vi "OscilloscopeDual.vi"() -> ()   [LabVIEW 2021]
uses:
  <userlib>/SciSDK/SciSDK_Labview.lvlib
panel:
  out "Digital CH3.3":i32[](graph)
  out "Digital CH3.2":i32[](graph)
  out "Digital CH3.1":i32[](graph)
  out "Digital CH3.0":i32[](graph)
  out "Digital CH2.3":i32[](graph)
  out "Digital CH2.2":i32[](graph)
  out "Digital CH2.1":i32[](graph)
  out "Digital CH2.0":i32[](graph)
  out "Digital CH1.3":i32[](graph)
  out "Digital CH1.2":i32[](graph)
  out "Digital CH1.1":i32[](graph)
  out "Digital CH1.0":i32[](graph)
  out "Digital CH0.3":i32[](graph)
  out "Digital CH0.2":i32[](graph)
  out "Digital CH0.1":i32[](graph)
  out "Analog CH1":dbl[](graph)
  out "Analog CH2":dbl[](graph)
  out "Analog CH3":dbl[](graph)
  out "Analog CH0":dbl[](graph)
  out "Digital CH0.0":i32[](graph)
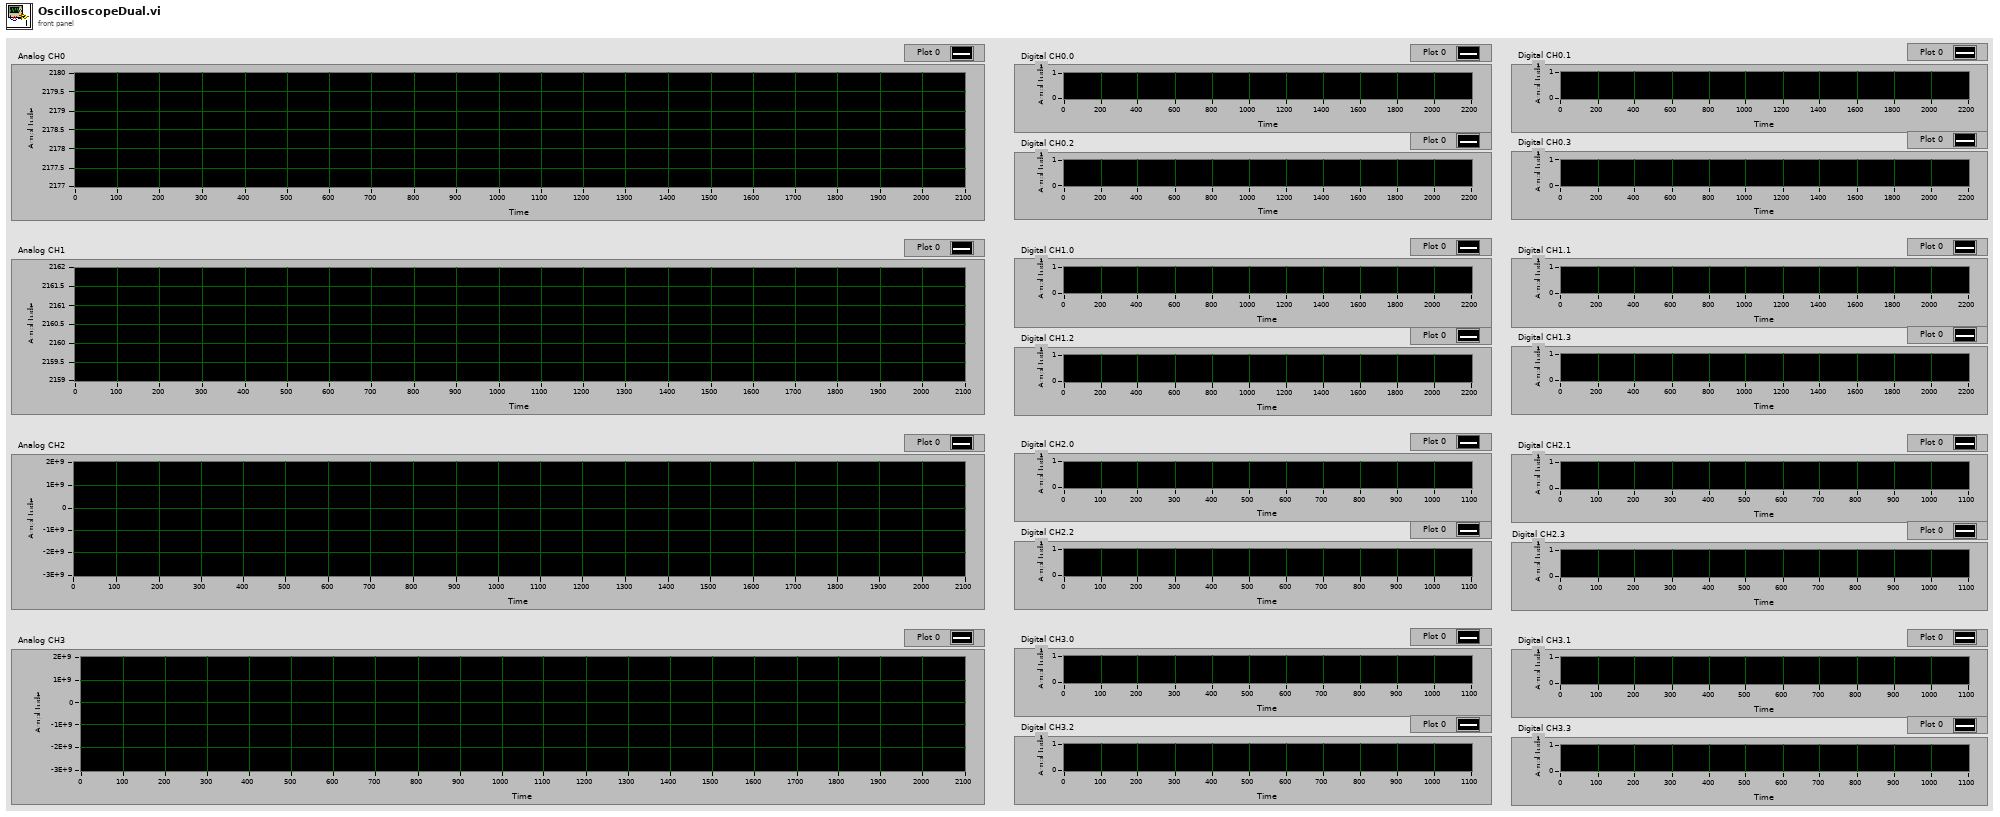
[diagram p1: front panel]
types:
  T1 = cluster{"Name":string, "Board Model":string, "Handle":u64}
  T2 = cluster{"Oscilloscope Dual Path":string, "Oscilloscope Dual Name":string}
  T3 = cluster{"Board Name":string, "Board Model":string, "Handle":u64}
  T4 = cluster{"magic":u32, "trigger_position":u32, "timecode":u32, "samples_analog":u32, "samples_digital":u32, "tracks_analog_per_channel":u32, "tracks_digital_per_channel":u32, "channels":u32, "analog":dbl[][], "digital_data":i32[][]}
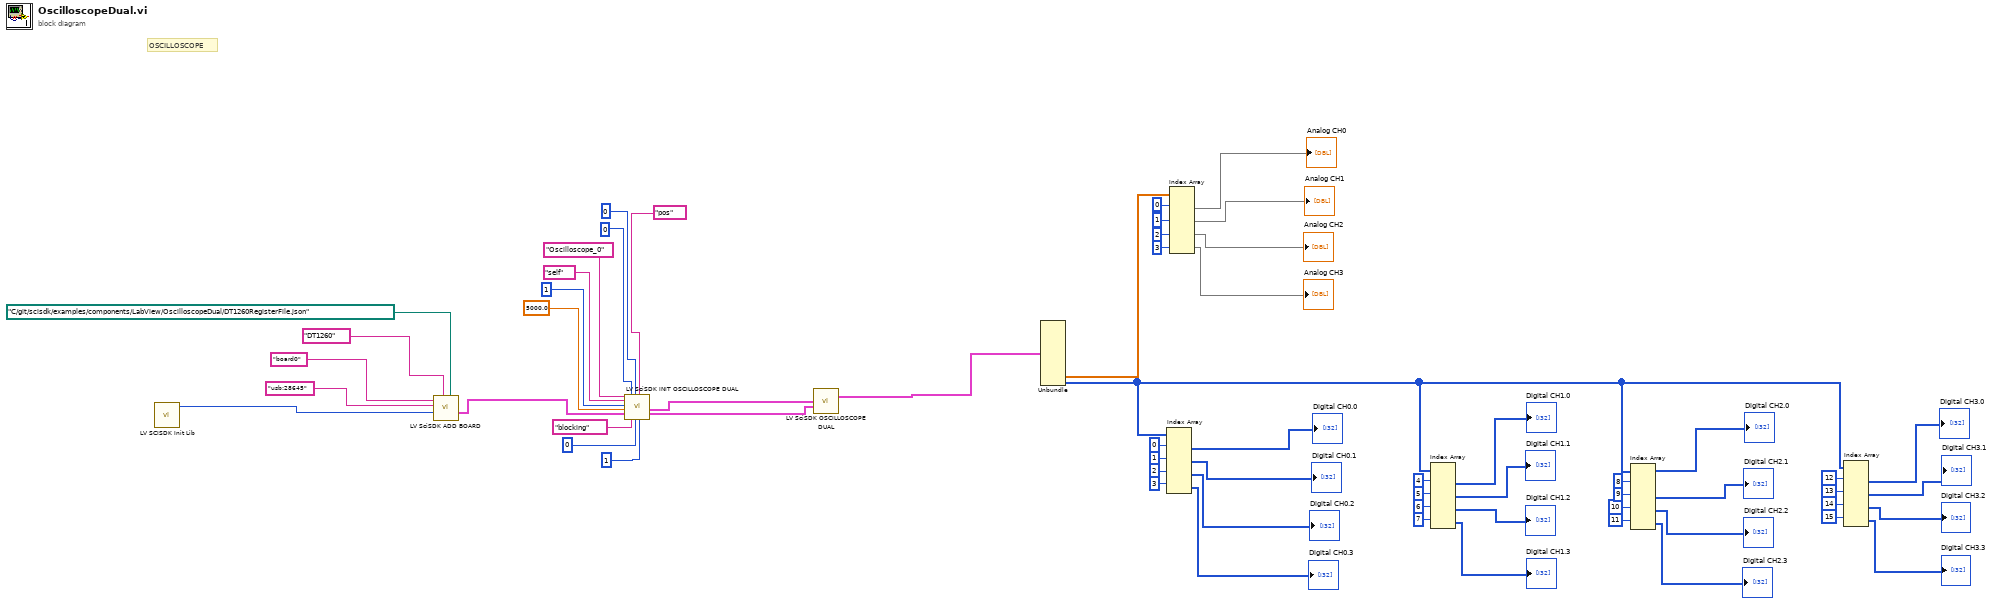
[diagram p0: block diagram]
diagram:
  # "OSCILLOSCOPE"
  n1 = call <userlib>:"LV SCISDK Init Lib.vi"() -> ("function return"=w19:u64)  [unwired: 11 in]
  n2 = call <userlib>:"LV SciSDK ADD BOARD.vi"("JsonFile"=path "C:/git/scisdk/examples/components/LabView/OscilloscopeDual/DT1260RegisterFile.json", "Board Model"="DT1260", "SciSDK Handle"=w19, "DevicePath"="usb:28645", "Name"="board0") -> ("Board Handle Out"=w11:T1)  [unwired: 4 in, 2 out]
  n3 = call <userlib>:"LV SciSDK INIT OSCILLOSCOPE DUAL.vi"("Oscilloscope Name"="Oscilloscope_0", "Trigger Mode"="self", "Decimator"=u32 1, "Timeout"=5000.0, "Board Handle In"=w11, "Pretrigger"=u32 0, "Acq Mode"="blocking", "Trigger Level"=u32 0, "Trigger Channel"=u32 0, "Trigger Polarity"="pos", "Auto Arm"=u32 1) -> ("Oscilloscope Dual Handle Out"=w1:T2, "Board Handle Out"=w2:T3)  [unwired: 6 in, 1 out]
  n4 = call <userlib>:"LV SciSDK OSCILLOSCOPE DUAL.vi"("Oscilloscope Dual Handle In"=w1, "Board Handle In"=w2) -> ("Oscilloscope Dual Buffer Out"=w3:T4)  [unwired: 9 in, 4 out]
  n5 = Unbundle(w3) -> ("analog"=w59:dbl[][], "digital_data"=w32:i32[][])  [unwired: 8 out]
  n6 = Index Array(array=w32, index (row) #1=0 ("index (row)"), index (row) #2=1 ("index (row)"), index (row) #3=2 ("index (row)"), index (row) #4=3 ("index (row)")) -> (element #1=→"Digital CH0.0":i32[], element #2=→"Digital CH0.1":i32[], element #3=→"Digital CH0.2":i32[], element #4=→"Digital CH0.3":i32[])  [unwired: 4 in]
  n7 = Index Array(array=w59, index (row) #1=0 ("index (row)"), index (row) #2=1 ("index (row)"), index (row) #3=2 ("index (row)"), index (row) #4=3 ("index (row)")) -> (element #1=→"Analog CH0":dbl[], element #2=→"Analog CH1":dbl[], element #3=→"Analog CH2":dbl[], element #4=→"Analog CH3":dbl[])  [unwired: 4 in]
  n8 = Index Array(array=w32, index (row) #1=4 ("index (row)"), index (row) #2=5 ("index (row)"), index (row) #3=6 ("index (row)"), index (row) #4=7 ("index (row)")) -> (element #1=→"Digital CH1.0":i32[], element #2=→"Digital CH1.1":i32[], element #3=→"Digital CH1.2":i32[], element #4=→"Digital CH1.3":i32[])  [unwired: 4 in]
  n9 = Index Array(array=w32, index (row) #1=8 ("index (row)"), index (row) #2=9 ("index (row)"), index (row) #3=10 ("index (row)"), index (row) #4=11 ("index (row)")) -> (element #1=→"Digital CH2.0":i32[], element #2=→"Digital CH2.1":i32[], element #3=→"Digital CH2.2":i32[], element #4=→"Digital CH2.3":i32[])  [unwired: 4 in]
  n10 = Index Array(array=w32, index (row) #1=12 ("index (row)"), index (row) #2=13 ("index (row)"), index (row) #3=14 ("index (row)"), index (row) #4=15 ("index (row)")) -> (element #1=→"Digital CH3.0":i32[], element #2=→"Digital CH3.1":i32[], element #3=→"Digital CH3.2":i32[], element #4=→"Digital CH3.3":i32[])  [unwired: 4 in]
